vi "database operating.vi"(5 "table name":string="CCID", 6 "Read or Write":enum16{"Read", "Write"}(ring), 8 "布尔":bool, 9 "SerNO":string="123456789012345678901234567", 10 "ID":string="24450", 11 "CCID":string="45132") -> (0 "SerNO OUT":string[](array[string]), 4 "OUTdata":string[][](array[string]), 7 "OUT MAXID":string)   [LabVIEW 2013]
uses:
  <vilib>/addons/database/Auxilliary.llb/DB Tools Column Info.ctl
  <vilib>/addons/database/Auxilliary.llb/DB Tools DataTypes.ctl
  <vilib>/addons/database/Connection.llb/DB Tools Open Connec (String).vi
  <vilib>/addons/database/Connection.llb/Conn Execute.vi
  <vilib>/addons/database/Recordset.llb/Rec Fetch Recordset Data (R).vi
  <vilib>/addons/database/Recordset.llb/Rec Destroy - Connection.vi
  <vilib>/addons/database/NI_Database_API.lvlib
panel:
  out "tables":string[](array[string])
  out "连接的字符串 2":string
  out "SerNO":string[][](array[string])
  out "MAXID":string[][](array[string])
  out "recordset data":variant[][](array[variant])
  out "连接的字符串":string
  out "日期/时间字符串":string
  in  "簇":T1
  in  "error in (no error)":errorcluster
  out "error out":errorcluster
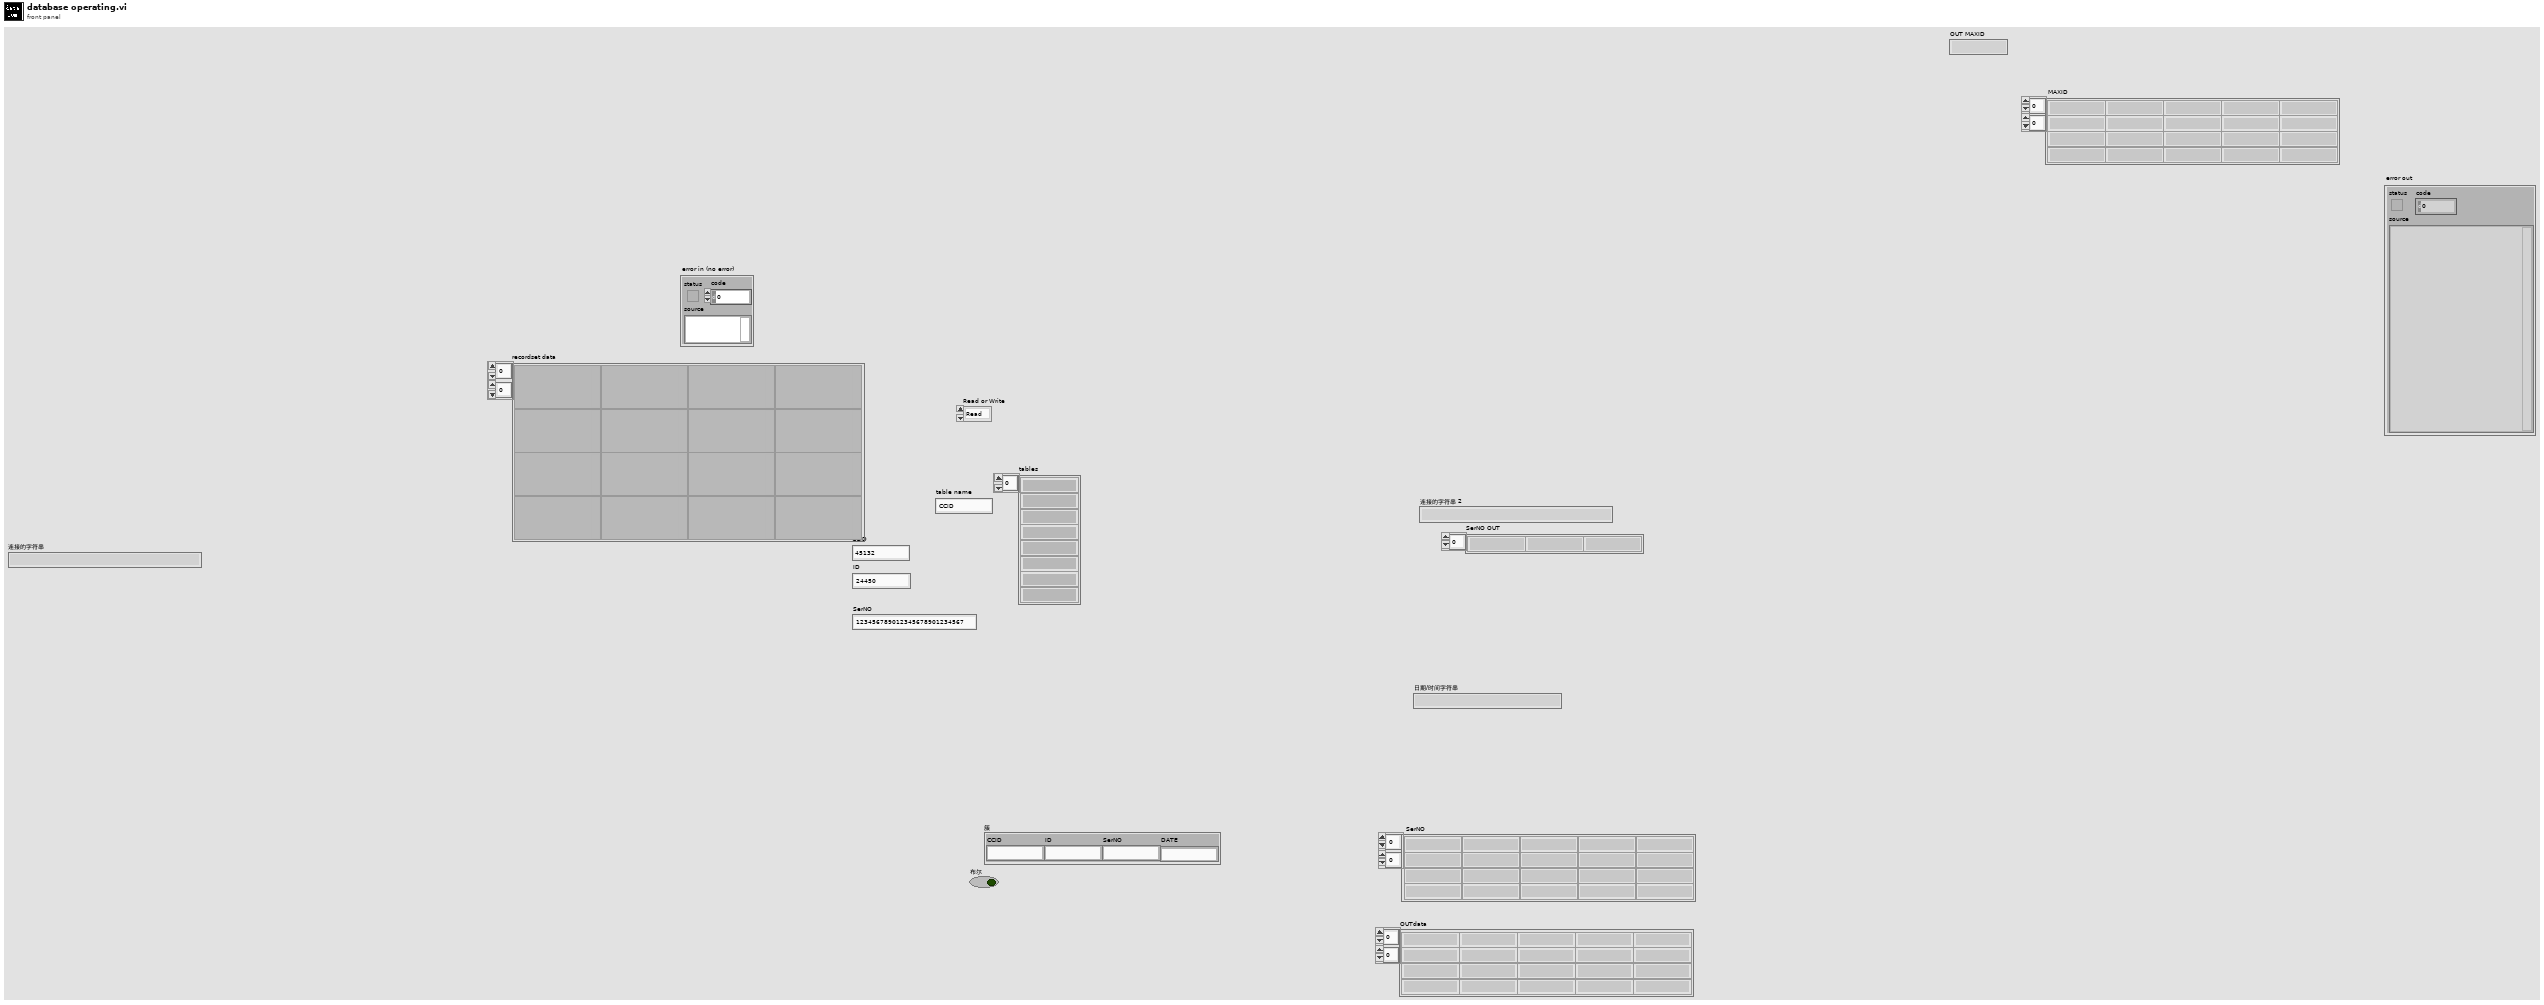
[diagram p1: front panel]
types:
  T1 = cluster{"CCID":string, "ID":string, "SerNO":string, "DATE":string}
  T2 = typedef "NI_Database_API.lvlib/DB Tools Column Info.ctl" = cluster{"column name":string, "data type":T3, "size":i32, "allow null?":bool}
  T3 = typedef "NI_Database_API.lvlib/DB Tools DataTypes.ctl" = enum16{"String", "Long (I32)", "Single (SGL)", "Double (DBL)", "Date/Time", "Binary"}
  T4 = typedef "NI_Database_API.lvlib/Conn ObjectReference.ctl" = refnum<k1>
  T5 = typedef "NI_Database_API.lvlib/Rec ObjectReference.ctl" = refnum<k1>
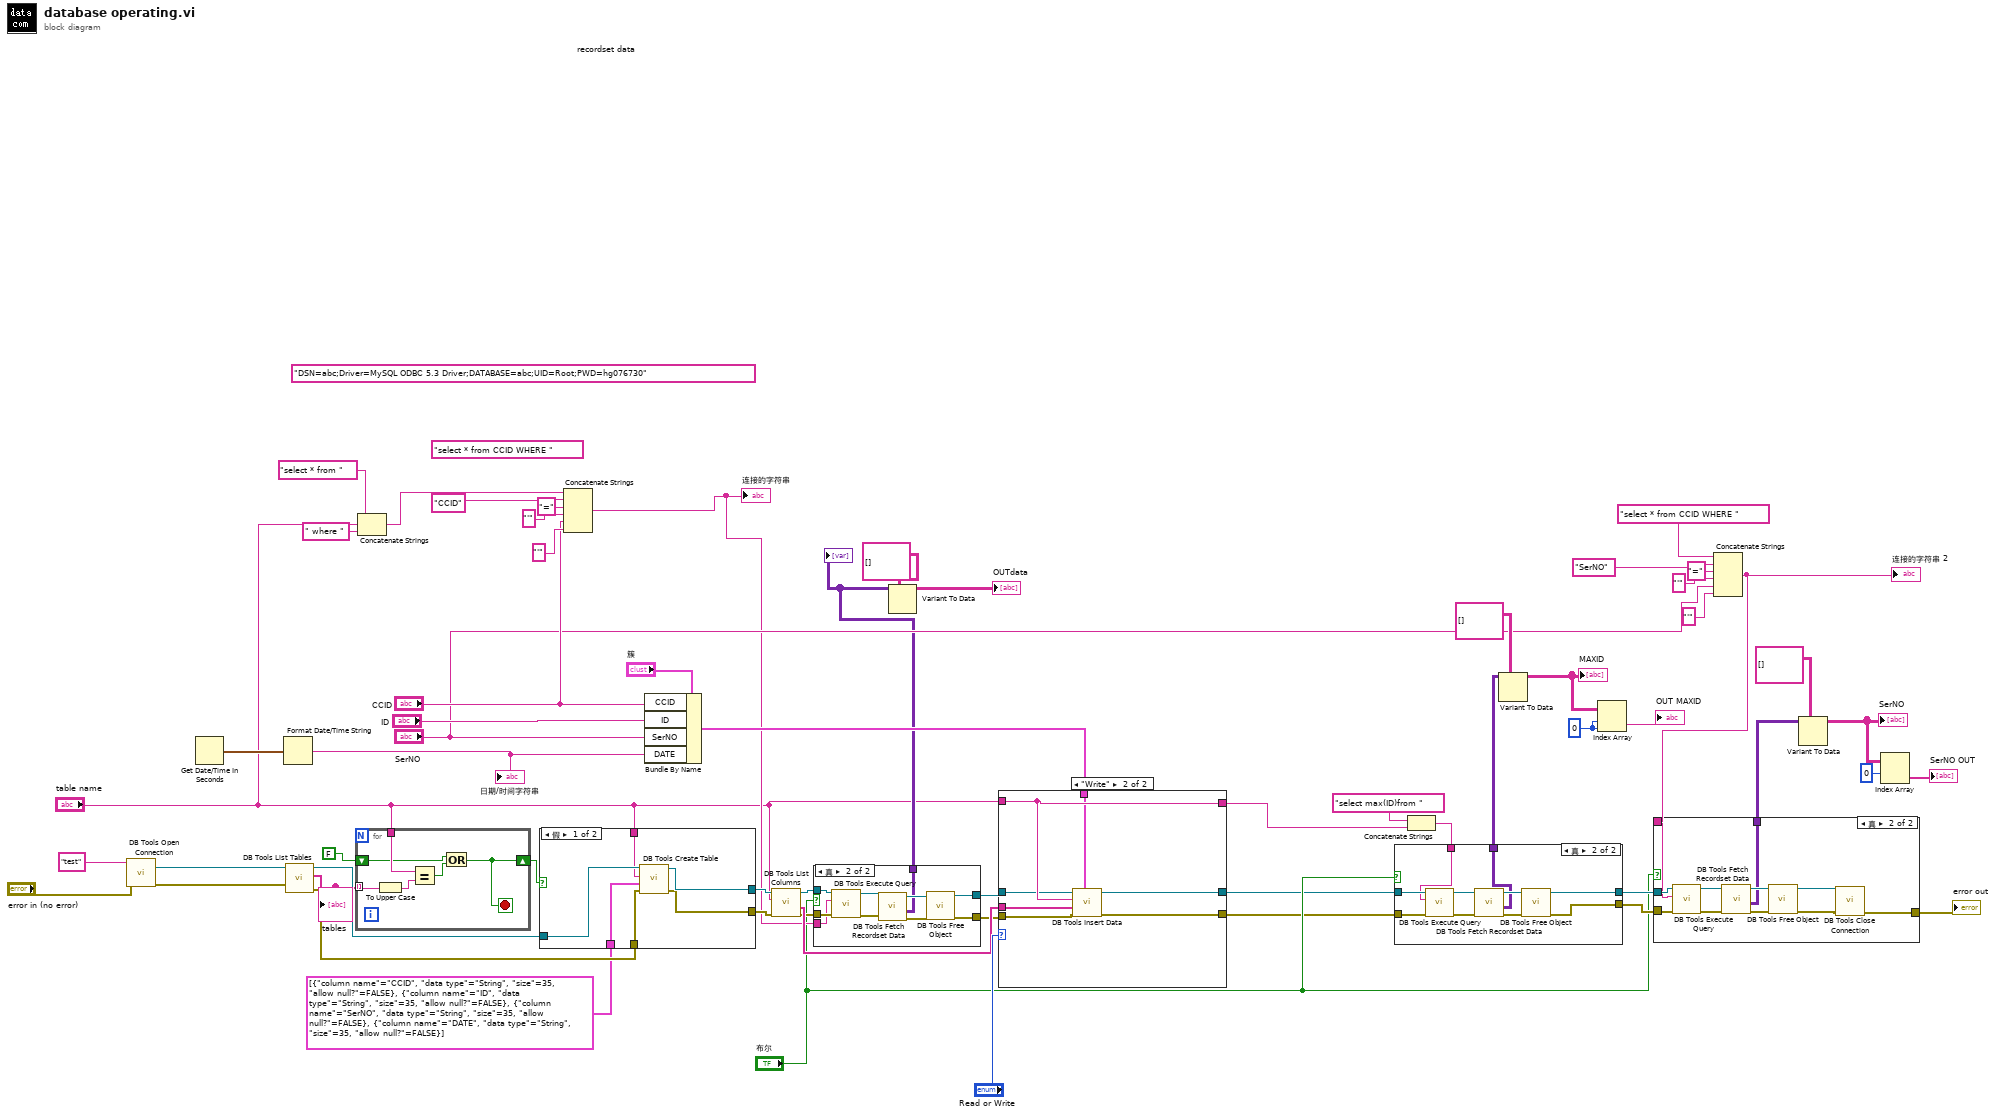
[diagram p0: block diagram]
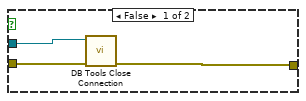
[diagram p3: hidden frame]
diagram:
  w33 = 0 ("禁用的索引 (列)")
  (unwired) "select * from CCID WHERE " ("字符串")
  (unwired) "DSN=abc;Driver=MySQL ODBC 5.3 Driver;DATABASE=abc;UID=Root;PWD=hg076730" ("userID")
  n1 = call-poly <vilib>:"DB Tools Open Connection.vi"("error in (no error)"="error in (no error)", "connection information"="test" ("table")) -> ("error out"=w54:errorcluster, "connection reference"=w55:T4)  [unwired: 6 in]
  n2 = Get Date/Time In Seconds() -> (seconds since 1Jan1904=w48:timestamp)
  n3 = Format Date/Time String(seconds (now)=w48) -> (date/time string=w47:string)  [unwired: 2 in]
  "日期/时间字符串" <- w47
  n4 = call <vilib>:"DB Tools List Tables.vi"("error in (no error)"=w54, "connection reference"=w55) -> ("error out"=w58:errorcluster, "tables"=w59:string[], "connection reference out"=w60:T4)  [unwired: 3 in]
  "tables" <- w59
  n5 = for {
    shift-right: [w65] -> w61
    shift-left: FALSE -> [w67]
    tunnel: w59 -> [w64] mode=indexing
    tunnel: "table name" -> [w68]
    stop <- w65 stop-if-true
    n6 = To Upper Case(1:w64) -> (0:w63:string)
    n7 = Equal?(x=w68, y=w63) -> (x = y?=w66:bool)
    n8 = Or(x=w67, y=w66) -> (x .or. y?=w65:bool)
  }
  n9 = Concatenate Strings("select * from " ("字符串"), "table name", " where " ("字符串")) -> (w5:string)
  n10 = case shown="假" w61 {
    tunnel: w60 -> [w74 w75]
    tunnel: w58 -> [w73 w76]
    tunnel: "table name" -> [w72 _]
    tunnel: [w71 w75] -> w57
    tunnel: [w70 w76] -> w56
    tunnel: T2[] [{"column name"="CCID", "data type"=enum."String", "size"=35, "allow null?"=FALSE}, {"column name"="ID", "data type"=enum."String", "size"=35, "allow null?"=FALSE}, {"column name"="SerNO", "data type"=enum."String", "size"=35, "allow null?"=FALSE}, {"column name"="DATE", "data type"=enum."String", "size"=35, "allow null?"=FALSE}] ("column information") -> [w69 _]
    frame False {
      n11 = call <vilib>:"DB Tools Create Table.vi"("error in (no error)"=w73, "column information"=w69, "table"=w72, "connection reference"=w74) -> ("error out"=w70:errorcluster, "connection reference out"=w71:T4)  [unwired: 4 in]
    }
    frame True {
    }
  }
  n12 = Concatenate Strings(w5, "CCID" ("字符串"), "=" ("字符串"), "'" ("字符串"), "CCID", "'" ("字符串")) -> (w13:string)
  "连接的字符串" <- w13
  n13 = Bundle By Name(cluster="簇", "CCID"="CCID", "ID"="ID", "SerNO"="SerNO", "DATE"=w47) -> (w49:T1)
  n14 = call <vilib>:"DB Tools List Columns.vi"("error in (no error)"=w56, "table"="table name", "connection reference"=w57) -> ("error out"=w16:errorcluster, "columns"=w45:string[], "connection reference out"=w14:T4)  [unwired: 1 in, 1 out]
  n15 = case shown="真" "布尔" {
    tunnel: [w78 w86] -> w17
    tunnel: w16 -> [w77 w85]
    tunnel: [w77 w82] -> w15
    tunnel: w14 -> [w78 w81]
    tunnel: w13 -> [_ w80]
    tunnel: [_ w79] -> w12
    frame False {
    }
    frame True {
      n16 = call-poly <vilib>:"DB Tools Execute Query.vi"("error in (no error)"=w85, "SQL query"=w80, "connection reference"=w81) -> ("error out"=w84:errorcluster, "recordset reference"=w88:T5)  [unwired: 5 in]
      n17 = call-poly <vilib>:"DB Tools Fetch Recordset Data.vi"("error in (no error)"=w84, "recordset reference"=w88) -> ("error out"=w83:errorcluster, "recordset data"=w79:variant[][], "recordset reference out"=w87:T5)  [unwired: 3 in]
      n18 = call-poly <vilib>:"DB Tools Free Object.vi"("error in (no error)"=w83, "recordset reference"=w87) -> ("error out"=w82:errorcluster, "connection reference"=w86:T4)  [unwired: 8 in]
    }
  }
  "recordset data" <- w12
  n19 = Variant To Data(type=string[][] [] ("数组"), Variant=w12) -> (data=→"OUTdata":string[][])  [unwired: 1 in, 1 out]
  n20 = case shown="\"Write\"" "Read or Write" {
    tunnel: "table name" -> [w90 w94]
    tunnel: w45 -> [_ w98]
    tunnel: [w89 w97] -> w9
    tunnel: w15 -> [w91 w96]
    tunnel: [w91 w95] -> w10
    tunnel: [w90 w94] -> w3
    tunnel: w17 -> [w89 w93]
    tunnel: w49 -> [_ w92]
    frame "Read", Default {
    }
    frame "Write" {
      n21 = call <vilib>:"DB Tools Insert Data.vi"("data"=w92, "error in (no error)"=w96, "columns"=w98, "table"=w94, "connection reference"=w93) -> ("error out"=w95:errorcluster, "connection reference out"=w97:T4)  [unwired: 5 in]
    }
  }
  n22 = Concatenate Strings("select max(ID)from " ("字符串"), w3) -> (w2:string)
  n23 = case shown="真" "布尔" {
    tunnel: w9 -> [w100 w106]
    tunnel: w10 -> [w99 w105]
    tunnel: w2 -> [_ w104]
    tunnel: [_ w103] -> w35
    tunnel: [w100 w102] -> w31
    tunnel: [w99 w101] -> w30
    frame False {
    }
    frame True {
      n24 = call-poly <vilib>:"DB Tools Execute Query.vi"("error in (no error)"=w105, "SQL query"=w104, "connection reference"=w106) -> ("error out"=w109:errorcluster, "recordset reference"=w110:T5)  [unwired: 5 in]
      n25 = call-poly <vilib>:"DB Tools Fetch Recordset Data.vi"("error in (no error)"=w109, "recordset reference"=w110) -> ("error out"=w108:errorcluster, "recordset data"=w103:variant[][], "recordset reference out"=w107:T5)  [unwired: 3 in]
      n26 = call-poly <vilib>:"DB Tools Free Object.vi"("error in (no error)"=w108, "recordset reference"=w107) -> ("error out"=w101:errorcluster, "connection reference"=w102:T4)  [unwired: 8 in]
    }
  }
  n27 = Variant To Data(type=string[][] [] ("数组"), Variant=w35) -> (data=w34:string[][])  [unwired: 1 in, 1 out]
  "MAXID" <- w34
  n28 = Index Array(array=w34, index (row)=w33, index (col)=w33) -> (element=→"OUT MAXID":string)
  n29 = Concatenate Strings("select * from CCID WHERE " ("字符串"), "SerNO" ("字符串"), "=" ("字符串"), "'" ("字符串"), "SerNO", "'" ("字符串")) -> (w22:string)
  "连接的字符串 2" <- w22
  n30 = case shown="真" "布尔" {
    tunnel: [w111 w124] -> w37
    tunnel: w31 -> [w113 w119]
    tunnel: w30 -> [w112 w118]
    tunnel: [_ w117] -> w28
    tunnel: w22 -> [_ w114]
    frame False {
      n31 = call <vilib>:"DB Tools Close Connection.vi"("error in (no error)"=w112, "connection reference"=w113) -> ("error out"=w111:errorcluster)  [unwired: 5 in]
    }
    frame True {
      n32 = call-poly <vilib>:"DB Tools Execute Query.vi"("error in (no error)"=w118, "SQL query"=w114, "connection reference"=w119) -> ("error out"=w122:errorcluster, "recordset reference"=w123:T5)  [unwired: 5 in]
      n33 = call-poly <vilib>:"DB Tools Fetch Recordset Data.vi"("error in (no error)"=w122, "recordset reference"=w123) -> ("error out"=w121:errorcluster, "recordset data"=w117:variant[][], "recordset reference out"=w120:T5)  [unwired: 3 in]
      n34 = call-poly <vilib>:"DB Tools Free Object.vi"("error in (no error)"=w121, "recordset reference"=w120) -> ("error out"=w115:errorcluster, "connection reference"=w116:T4)  [unwired: 8 in]
      n35 = call <vilib>:"DB Tools Close Connection.vi"("error in (no error)"=w115, "connection reference"=w116) -> ("error out"=w124:errorcluster)  [unwired: 5 in]
    }
  }
  "error out" <- w37
  n36 = Variant To Data(type=string[][] [] ("数组"), Variant=w28) -> (data=w20:string[][])  [unwired: 1 in, 1 out]
  "SerNO" <- w20
  n37 = Index Array(array=w20, index (row)=0 ("索引 (行)")) -> (element=→"SerNO OUT":string[])  [unwired: 1 in]
